vi "Read.vi"(1 "R_Channel":string="0", 2 "R_Call_Function":string="outputMeasurementSenseVoltage", 3 "IP":string="192.168.0.250") -> (0 "R_Return":string)   [LabVIEW 2018]
panel:
  out "Full  Command":string
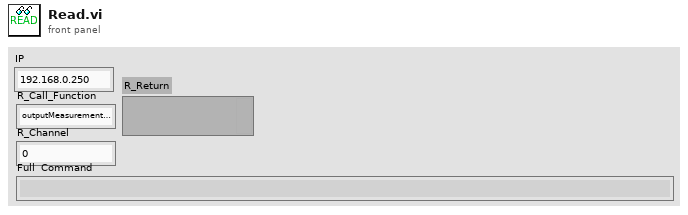
[diagram p1: front panel]
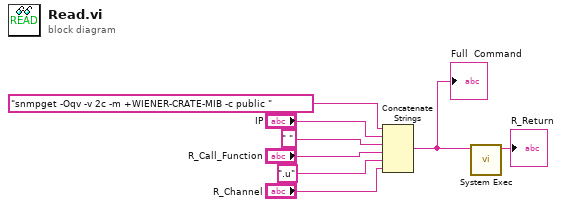
[diagram p0: block diagram]
diagram:
  n1 = Concatenate Strings("snmpget -Oqv -v 2c -m +WIENER-CRATE-MIB -c public ", "IP", " ", "R_Call_Function", ".u", "R_Channel") -> (w2:string)
  "Full  Command" <- w2
  n2 = call <vilib>:"System Exec.vi"("command line"=w2) -> ("standard output"=→"R_Return":string)  [unwired: 7 in, 3 out]
